vi "OpenProject.vi"(11 "Array":string[](array[string])) -> (2 "source":string, 3 "code":i32)   [LabVIEW 2020]
uses:
  <vilib>/addons/_JKI Toolkits/Caraya/run-tests/Run Test (ProjectRefnum).vi
  <vilib>/addons/_JKI Toolkits/Caraya/Caraya.lvlib
  <vilib>/addons/_JKI Toolkits/Caraya/classes/Test Suite/Test Suite.lvclass
  <vilib>/addons/_JKI Toolkits/Caraya/classes/Test Report/Test Report.lvclass
  <vilib>/PNR/Caraya JUnit for Azure Pipelines/JUnit for Azure Pipelines/JUnit for Azure Pipelines.lvclass
  <vilib>/addons/_JKI Toolkits/Caraya/classes/Test Runner.Folder/Test Runner.Folder.lvclass
  <vilib>/addons/_JKI Toolkits/Caraya/classes/Test Runner/Test Runner.lvclass
  C:/Program Files/National Instruments/LabVIEW 2020/vi.lib/addons/_JKI Toolkits/Caraya/classes/Test Runner/Test Runner.lvclass
  C:/Program Files/National Instruments/LabVIEW 2020/vi.lib/addons/_JKI Toolkits/Caraya/classes/Test Report/Test Report.lvclass
panel:
  out "path":path
  out "Error out":errorcluster
  in  "Error_In":errorcluster
  # "Opens the Project file"
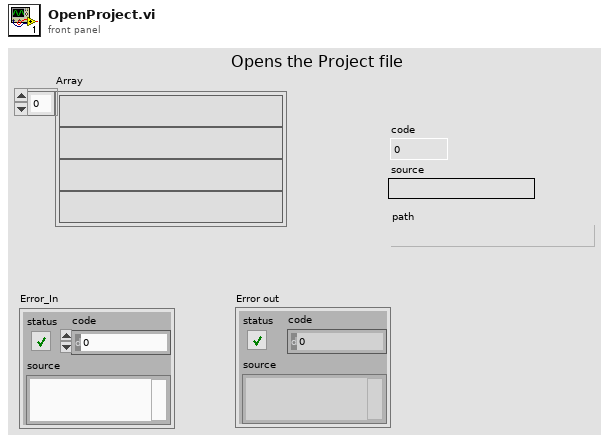
[diagram p1: front panel]
types:
  T1 = enum32{"Invalid", "Standard", "Closed", "Hidden", "Minimized", "Maximized"}
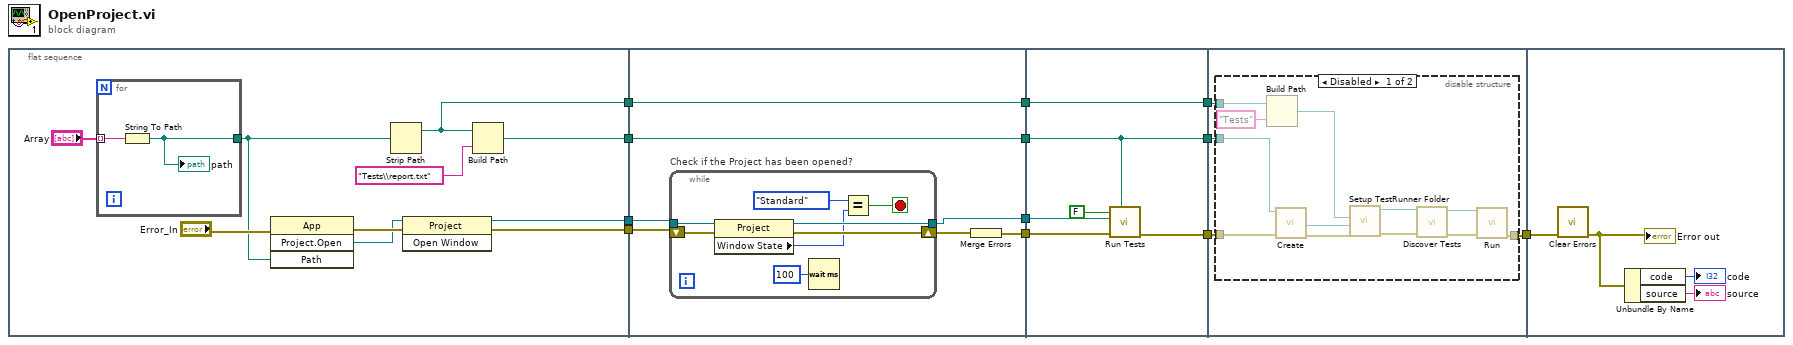
[diagram p0: block diagram]
diagram:
  n1 = flat-sequence {
    tunnel: [w20] -> w12
    tunnel: [w19] -> w11
    tunnel: [w14] -> w7
    tunnel: [w13] -> w2
    tunnel: w12 -> [w31]
    tunnel: w11 -> [w30]
    tunnel: [w28] -> w10
    tunnel: [w27] -> w9
    tunnel: [w26] -> w8
    tunnel: w7 -> [w26]
    tunnel: [w25] -> w3
    tunnel: w2 -> [w25]
    tunnel: [w44] -> w6
    tunnel: w10 -> [w43]
    tunnel: w9 -> [w45]
    tunnel: w8 -> [w40]
    tunnel: [w41] -> w4
    tunnel: w3 -> [w41]
    tunnel: [w40] -> w1
    tunnel: w6 -> [w49]
    tunnel: [w47] -> w5
    tunnel: w4 -> [w46]
    tunnel: w1 -> [w48]
    tunnel: w5 -> [w62]
    frame #0 {
      n2 = for {
        tunnel: [w24] -> w16
        tunnel: "Array" -> [w23] mode=indexing
        n3 = String To Path(string=w23) -> (path=w24:path)
        "path" <- w24
      }
      n4 = invoke class="App" method="Project.Open"(error in="Error_In", "Path"=w16) -> (error out=w22:errorcluster, "Project:Open"=w21:refnum<vi>)  [unwired: 2 in, 2 out]
      n5 = Strip Path(path=w16) -> (stripped path=w13:path)  [unwired: 1 out]
      n6 = invoke class="Project" method="Open Window"(reference=w21, error in=w22) -> (reference out=w19:refnum<vi>, error out=w20:errorcluster)  [unwired: 1 in, 1 out]
      n7 = Build Path(base path=w13, name or relative path="Tests\\report.txt") -> (appended path=w14:path)
    }
    frame #1 {
      n8 = while "Check if the Project has been opened?" {
        tunnel: [w37] -> w27
        shift-right: [w38] -> w29
        shift-left: w31 -> [w33]
        tunnel: w30 -> [w32]
        stop <- w34 stop-if-true
        n9 = property class="Project"(reference=w32, error in=w33) -> (reference out=w37:refnum<vi>, error out=w38:errorcluster, "Window State"=w36:T1)
        n10 = Wait (ms)(milliseconds to wait=u32 100) -> ()  [unwired: 1 out]
        n11 = Equal?(x=T1."Standard" ("Window State 2"), y=w36) -> (x = y?=w34:bool)
      }
      n12 = Merge Errors(w29) -> (w28:errorcluster)
    }
    frame #2 {
      n13 = call-poly <vilib>:"Run Tests.vi"("Report Path"=w40, "error in"=w43, "Project Refnum"=w45, "Interactive (T)"=FALSE) -> ("error out"=w44:errorcluster)  [unwired: 6 in, 1 out]
    }
    frame #3 {
      n14 = disable-structure shown="Disabled" {
        disable-tunnel: w49 -> [w61 _]
        disable-tunnel: w48 -> [w57 _]
        disable-tunnel: [w52 _] -> w47
        disable-tunnel: w46 -> [w51 _]
        frame Disabled {
          n15 = Build Path(base path=w51, name or relative path="Tests") -> (appended path=w50:path)
          n16 = call <vilib>:"Create.vi"("error in (no error)"=w61, "Path"=w57) -> ("error out"=w60:errorcluster, "JUnit for Azure Pipelines"=w59:refnum<class "JUnit for Azure Pipelines.lvclass">)  [unwired: 8 in]
          n17 = call <vilib>:"Setup TestRunner Folder.vi"("error in (no error)"=w60, "Test Report"=w59, "Directory to search"=w50) -> ("error out"=w56:errorcluster, "Test Runner.Folder out"=w55:refnum<class "Test Runner.Folder.lvclass">)  [unwired: 7 in]
          n18 = call <vilib>:"Discover Tests.vi"("error in (no error)"=w56, "Test Runner in"=w55) -> ("error out"=w54:errorcluster, "Test Runner out"=w53:refnum<class "Test Runner.Folder.lvclass">)  [unwired: 8 in]
          n19 = call <vilib>:"Run.vi"("error in (no error)"=w54, "Test Runner in"=w53) -> ("error out"=w52:errorcluster)  [unwired: 7 in, 2 out]
        }
        frame Enabled {
        }
      }
    }
    frame #4 {
      n20 = call <vilib>:"Clear Errors.vi"("error in (no error)"=w62) -> ("error out"=w63:errorcluster)  [unwired: 5 in, 1 out]
      "Error out" <- w63
      n21 = Unbundle By Name(w63) -> ("code"=→"code":i32, "source"=→"source":string)
    }
  }
